vi "FTW-Test-MessagePipe.vi"() -> (0 "Test Result":errorcluster)   [LabVIEW 2015]
uses:
  src/core/type/FTW-Type-JSON.ctl
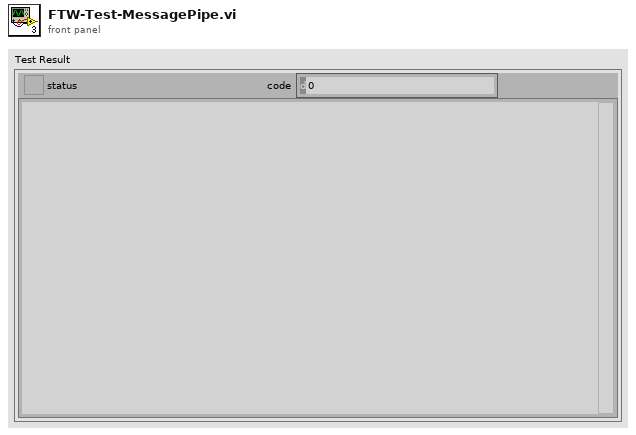
[diagram p1: front panel]
types:
  T1 = typedef "FTW-Type-JSON.ctl" = refnum<data-value>
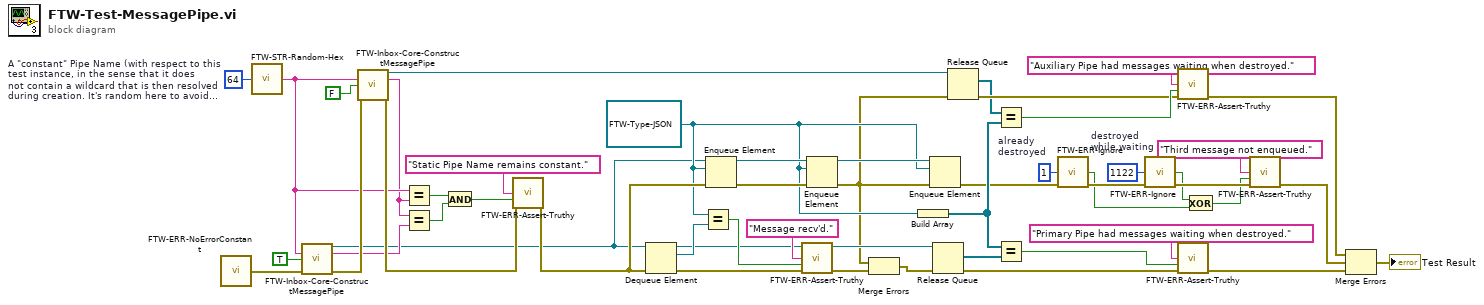
[diagram p0: block diagram]
diagram:
  w6 = 1  # already destroyed
  w12 = 1122  # destroyed while waiting
  w25 = T1 refnum ("element")
  w46 = 64  # A "constant" Pipe Name (with respect to this test instance, in the sense that it does not contain a wildcard that is then resolved during creation. It's random here to avoid collision with other instances of this test running in parallel.)
  n1 = call "FTW-ERR-NoErrorConstant.vi"() -> ("no error"=w47:errorcluster)
  n2 = call "FTW-STR-Random-Hex.vi"("String Length"=w46) -> ("Random Hex String"=w41:string)  [unwired: 3 in]
  n3 = call "FTW-Inbox-Core-ConstructMessagePipe.vi"("Actor Identity (empty to create unnamed actor)"=w41, "Is Primary?"=TRUE, "error in"=w47) -> ("Message Pipe"=w23:refnum<queue>, "Resolved Actor Identity"=w42:string, "error out"=w44:errorcluster)  [unwired: 10 in]
  n4 = call "FTW-Inbox-Core-ConstructMessagePipe.vi"("Actor Identity (empty to create unnamed actor)"=w41, "Is Primary?"=FALSE, "error in"=w44) -> ("Message Pipe"=w22:refnum<queue>, "Resolved Actor Identity"=w34:string, "error out"=w50:errorcluster)  [unwired: 10 in]
  n5 = Equal?(x=w41, y=w34) -> (x = y?=w40:bool)
  n6 = Equal?(x=w34, y=w42) -> (x = y?=w33:bool)
  n7 = And(x=w40, y=w33) -> (x .and. y?=w39:bool)
  n8 = call "FTW-ERR-Assert-Truthy.vi"("Assertion"="Static Pipe Name remains constant.", "Assertion holds true?"=w39, "error in"=w50) -> ("error out"=w49:errorcluster)  [unwired: 12 in]
  n9 = Dequeue Element(queue=w23, error in (no error)=w49) -> (queue out=w27:refnum<queue>, element=w32:T1, error out=w29:errorcluster)  [unwired: 1 in, 1 out]
  n10 = Equal?(x=w25, y=w32) -> (x = y?=w30:bool)
  n11 = Enqueue Element(queue=w23, element=w25, error in (no error)=w49) -> (queue out=w37:refnum<queue>, error out=w36:errorcluster)  [unwired: 1 in, 1 out]
  n12 = call "FTW-ERR-Assert-Truthy.vi"("Assertion"="Message recv'd.", "Assertion holds true?"=w30, "error in"=w29) -> ("error out"=w28:errorcluster)  [unwired: 12 in]
  n13 = Enqueue Element(queue=w37, element=w25, error in (no error)=w36) -> (queue out=w35:refnum<queue>, error out=w21:errorcluster)  [unwired: 1 in, 1 out]
  n14 = Merge Errors(w21, w28) -> (w26:errorcluster)
  n15 = Build Array(w25) -> (w15:T1[])
  n16 = Enqueue Element(queue=w35, element=w25, error in (no error)=w21) -> (error out=w5:errorcluster)  [unwired: 1 in, 2 out]
  n17 = Release Queue(queue=w27, error in (no error)=w26) -> (remaining elements=w17:T1[], error out=w9:errorcluster)  [unwired: 1 in, 1 out]
  n18 = Release Queue(queue=w22, error in (no error)=w21) -> (remaining elements=w16:T1[], error out=w18:errorcluster)  [unwired: 1 in, 1 out]
  n19 = Equal?(x=w16, y=w15) -> (x = y?=w20:bool)
  n20 = Equal?(x=w15, y=w17) -> (x = y?=w24:bool)
  n21 = call "FTW-ERR-Ignore.vi"("Error Code"=w6, "error in"=w5) -> ("Error Cleared?"=w2:bool, "error out"=w4:errorcluster)  [unwired: 12 in]
  n22 = call "FTW-ERR-Ignore.vi"("Error Code"=w12, "error in"=w4) -> ("Error Cleared?"=w3:bool, "error out"=w11:errorcluster)  [unwired: 12 in]
  n23 = call "FTW-ERR-Assert-Truthy.vi"("Assertion"="Auxiliary Pipe had messages waiting when destroyed.", "Assertion holds true?"=w20, "error in"=w18) -> ("error out"=w14:errorcluster)  [unwired: 12 in]
  n24 = call "FTW-ERR-Assert-Truthy.vi"("Assertion"="Primary Pipe had messages waiting when destroyed.", "Assertion holds true?"=w24, "error in"=w9) -> ("error out"=w8:errorcluster)  [unwired: 12 in]
  n25 = Exclusive Or(1:w2, 2:w3) -> (0:w1:bool)
  n26 = call "FTW-ERR-Assert-Truthy.vi"("Assertion"="Third message not enqueued.", "Assertion holds true?"=w1, "error in"=w11) -> ("error out"=w10:errorcluster)  [unwired: 12 in]
  n27 = Merge Errors(w14, w10, w8) -> (→"Test Result":errorcluster)
